vi "LabVIEW host computer v4.0.vi"() -> ()   [LabVIEW 2018]
uses:
  <vilib>/Instr/_visa.llb/VISA Configure Serial Port (Instr).vi
  <vilib>/regexp/Match Regular Expression.xnode
panel:
  out "HydrogenRemoteData":string="INSERT INTO MonitoringData(time, temperature, humidity)\nVALUES('2020/10/9 17:58:35', 24, 69)"
  in  "ConnectionString":string="DSN=myDB;"
  in  "选项卡控件":enum32{"双通道功率 ", "氢气浓度"}(tab)
  in  "选项卡控件 2":enum32{"通讯设置/数据显示"}(tab)
  in  "Reset":bool
  out "?":string
  in  "VISA resource name":refnum<visa-resource-name> caption="选择串口"
  in  "baud rate (9600)":u32=9600 caption="波特率"
  out "CH1 power":dbl
  out "?":string
  out "CH2 power":dbl
  out "CH1/CH2":dbl
  out "氢气浓度 4":dbl
  out "CH1 Power 2":dbl(graph)
  out "CH2 Power 2":dbl(graph)
  out "氢气浓度":dbl(graph)
  out "氢气浓度":dbl[](graph)
  in  "氢气输入":dbl[](array[numeric])
  out "氢气变化波长":dbl
  out "氢气浓度 3":dbl
  out "标定X":dbl[](array[numeric])
  out "氢气浓度 2":dbl
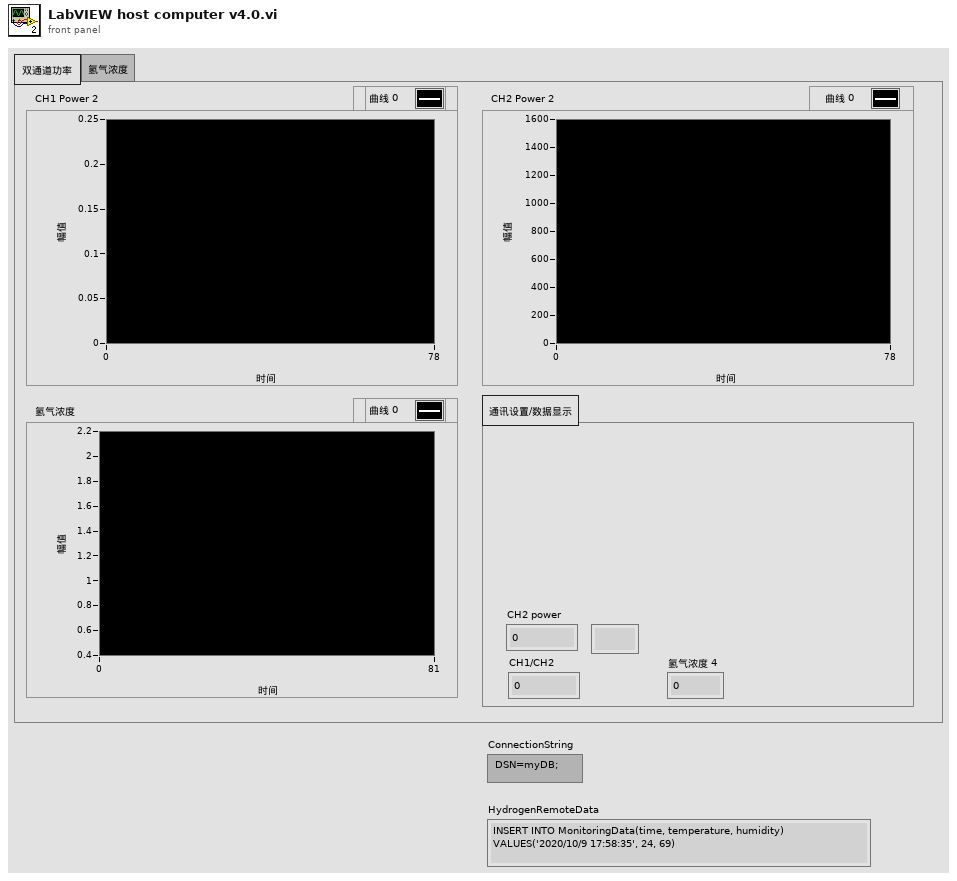
[diagram p1: front panel]
types:
  T1 = enum16{"open", "replace", "create", "open or create", "replace or create", "replace or create with confirmation"}
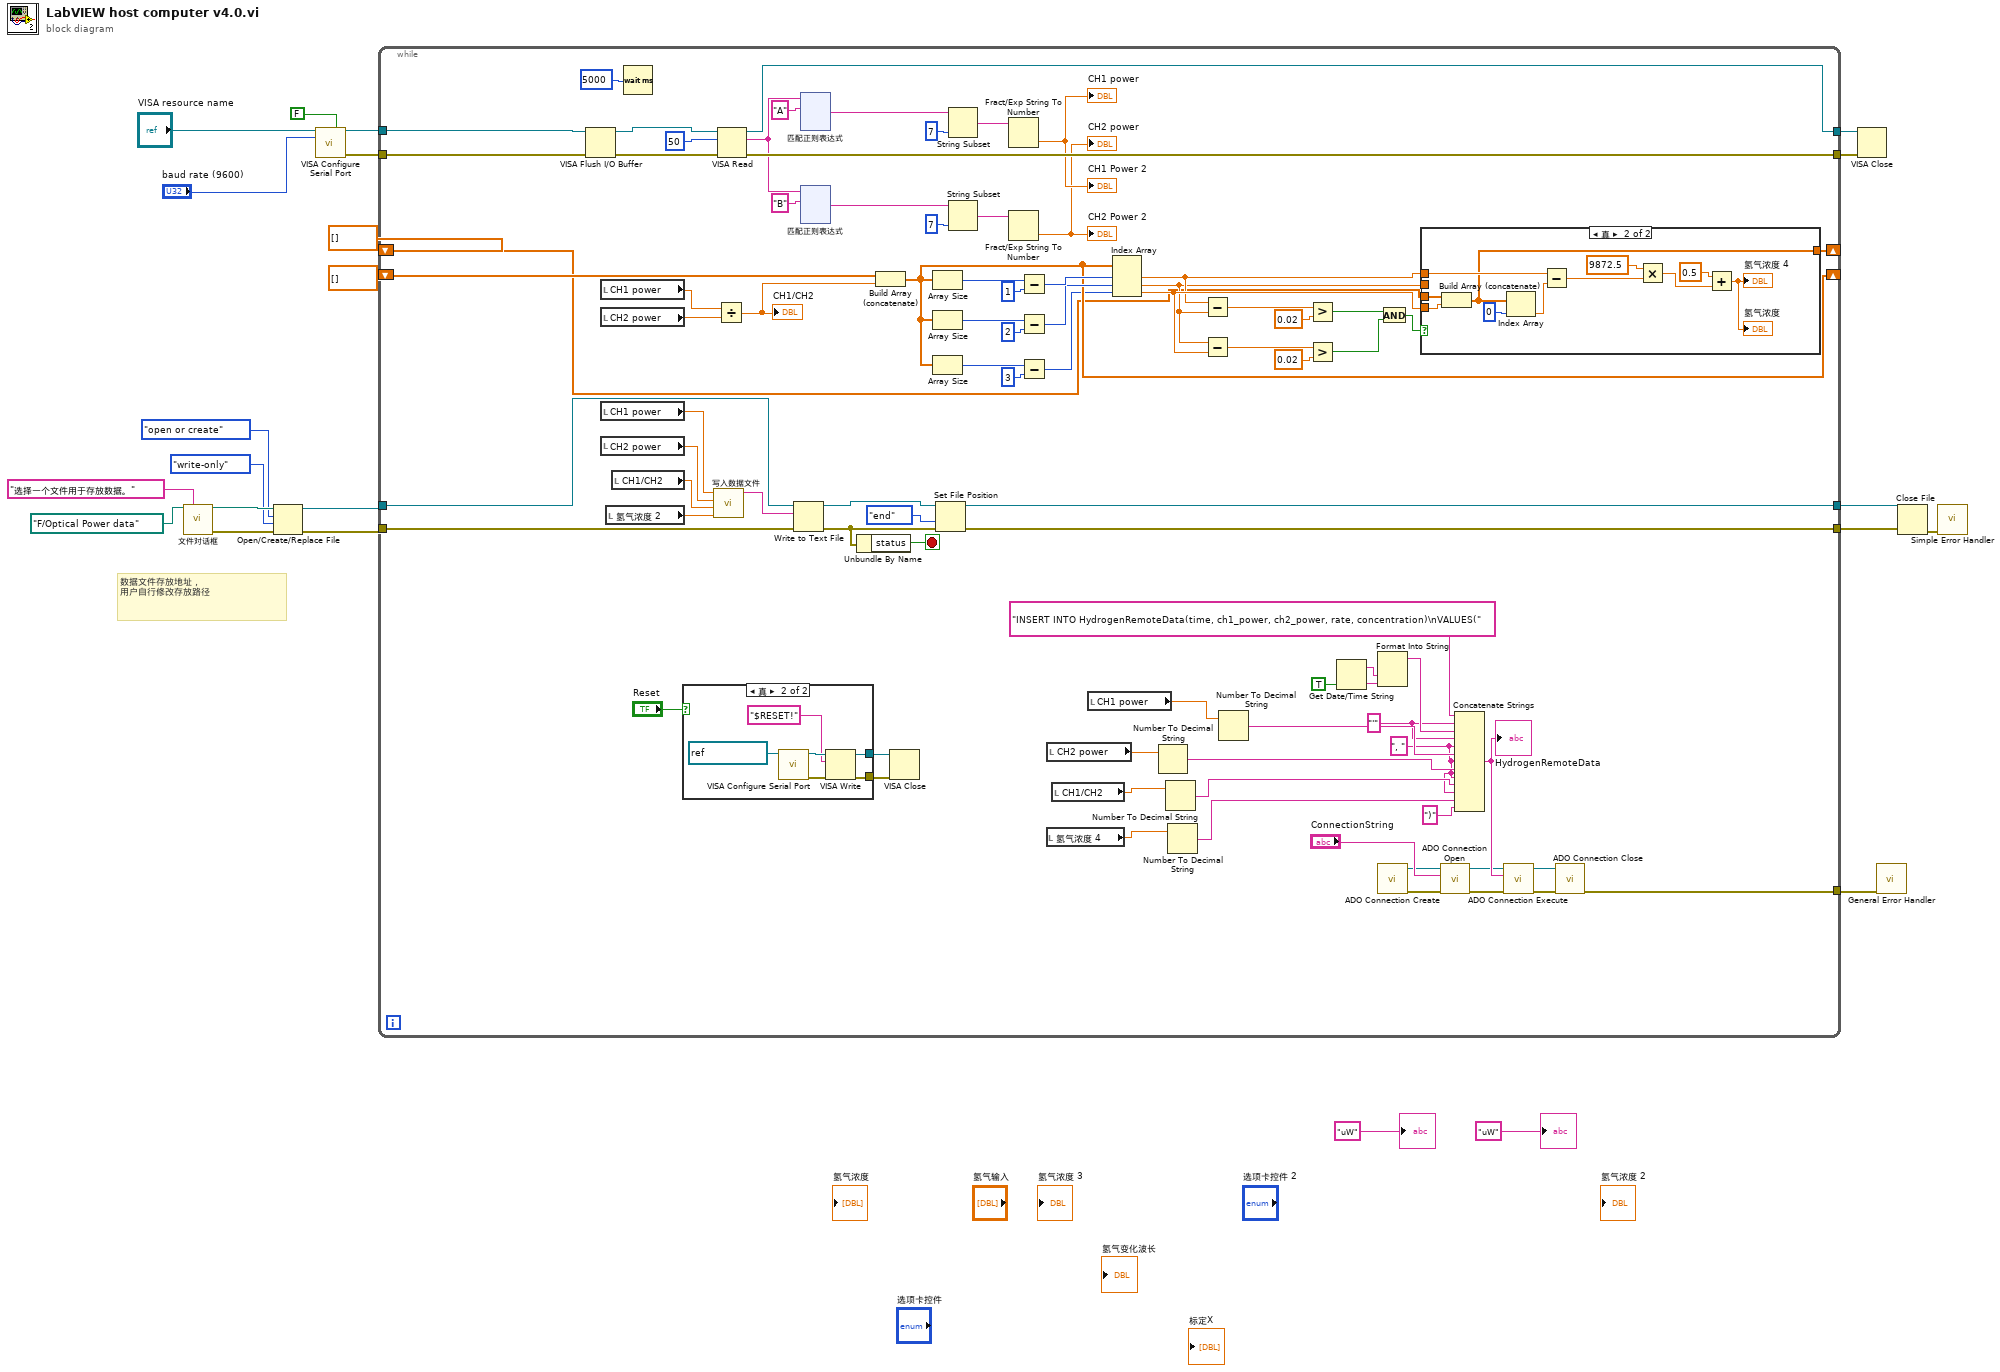
[diagram p0: block diagram]
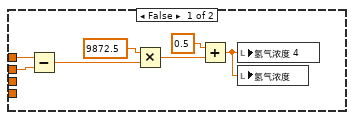
[diagram p3: hidden frame]
diagram:
  # "数据文件存放地址，\n用户自行修改存放路径"
  n1 = call "文件对话框"("start path"=path "F:/Optical Power data", "prompt"="选择一个文件用于存放数据。") -> ("selected path"=w15:path, "error out"=w14:errorcluster)  [unwired: 10 in, 2 out]
  n2 = Open/Create/Replace File(file path (use dialog)=w15, error in=w14, operation (0:open)=T1."open or create" ("操作(0:open)"), access (0:read/write)=enum16{"read/write", "read-only", "write-only"}."write-only" ("权限(0:read/write)")) -> (refnum out=w10:refnum<file>, error out=w9:errorcluster)  [unwired: 2 in, 1 out]
  n3 = call-poly "VISA Configure Serial Port"("VISA resource name"="VISA resource name", "Enable Termination\nChar (T)"=FALSE ("Enable Termination\nChar (T)"), "baud rate (9600)"="baud rate (9600)") -> ("VISA resource name out"=w20:refnum<visa-resource-name>, "error out"=w19:errorcluster)  [unwired: 11 in]
  n4 = while {
    tunnel: w20 -> [w108]
    tunnel: w19 -> [w107]
    tunnel: [w104] -> w18
    tunnel: w10 -> [w88]
    tunnel: w9 -> [w87]
    tunnel: [w86] -> w8
    tunnel: [w85] -> w7
    tunnel: [w84] -> w6
    shift-right: [w63] -> _
    shift-left: dbl[] [] -> [w68]
    shift-right: [w52] -> _
    shift-left: dbl[] [] -> [w53]
    tunnel: [w24] -> w1
    stop <- w89 stop-if-true
    w28 = ", " ("字符串")
    w34 = "'" ("字符串")
    n5 = VISA Flush I/O Buffer(VISA resource name=w108, error in (no error)=w107) -> (VISA resource name out=w106:refnum<visa-resource-name>, error out=w105:errorcluster)  [unwired: 1 in]
    n6 = local read "CH1 power"() -> (w78:dbl)
    n7 = local read "CH2 power"() -> (w77:dbl)
    n8 = local read "CH1 power"() -> (w93:dbl)
    n9 = local read "CH2 power"() -> (w94:dbl)
    n10 = local read "氢气浓度 2"() -> (w96:dbl)
    n11 = local read "CH1/CH2"() -> (w95:dbl)
    n12 = Wait (ms)(milliseconds to wait=u32 5000 ("毫秒计时值")) -> ()  [unwired: 1 out]
    n13 = case shown="真" "Reset" {
      tunnel: [_ w112] -> w50
      tunnel: [_ w111] -> w49
      frame False {
      }
      frame True {
        n14 = call-poly "VISA Configure Serial Port"("VISA resource name"=refnum<visa-resource-name> "COM3") -> ("VISA resource name out"=w114:refnum<visa-resource-name>, "error out"=w110:errorcluster)  [unwired: 13 in]
        n15 = VISA Write(VISA resource name=w114, write buffer="$RESET!" ("写入缓冲区"), error in (no error)=w110) -> (VISA resource name out=w112:refnum<visa-resource-name>, error out=w111:errorcluster)  [unwired: 1 out]
      }
    }
    n16 = call "写入数据文件.vi"("氢气浓度 2"=w96, "CH1/CH2"=w95, "CH2 Power"=w94, "CH1 Power"=w93) -> ("连接的字符串"=w97:string)  [unwired: 7 in]
    n17 = Divide(x=w78, y=w77) -> (x/y=w69:dbl)
    "CH1/CH2" <- w69
    n18 = VISA Read(VISA resource name=w106, byte count=u32 50 ("字节总数"), error in (no error)=w105) -> (VISA resource name out=w86:refnum<visa-resource-name>, read buffer=w83:string, error out=w104:errorcluster)  [unwired: 1 out]
    n19 = Write to Text File(file (use dialog)=w88, text=w97, error in=w87) -> (refnum out=w90:refnum<file>, error out=w91:errorcluster)  [unwired: 1 in, 1 out]
    n20 = xnode "匹配正则表达式"("输入字符串"=w83, "正则表达式"="A") -> ("匹配之后"=w102:string)  [unwired: 4 in, 4 out]
    n21 = xnode "匹配正则表达式"("输入字符串"=w83, "正则表达式"="B") -> ("匹配之后"=w98:string)  [unwired: 4 in, 4 out]
    n22 = Unbundle By Name(w91) -> ("status"=w89:bool)
    n23 = Build Array (concatenate)(w68, w69) -> (w63:dbl[])
    n24 = VISA Close(VISA resource name=w50, error in (no error)=w49) -> ()  [unwired: 1 out]
    n25 = Array Size(array=w63) -> (size(s)=w75:i32)
    n26 = Array Size(array=w63) -> (size(s)=w72:i32)
    n27 = Array Size(array=w63) -> (size(s)=w65:i32)
    n28 = Set File Position(refnum=w90, from (0:start)=enum16{"start", "end", "current"}."end" ("自（0:起始）"), error in=w91) -> (refnum out=w85:refnum<file>, error out=w84:errorcluster)  [unwired: 1 in]
    n29 = String Subset(string=w102, length (rest)=7 ("长度（剩余）")) -> (substring=w82:string)  [unwired: 1 in]
    n30 = String Subset(string=w98, length (rest)=7 ("长度（剩余）")) -> (substring=w80:string)  [unwired: 1 in]
    n31 = Fract/Exp String To Number(string=w82) -> (number=→"CH1 Power 2" →"CH1 power":dbl)  [unwired: 3 in, 1 out]
    n32 = Fract/Exp String To Number(string=w80) -> (number=→"CH2 Power 2" →"CH2 power":dbl)  [unwired: 3 in, 1 out]
    n33 = Subtract(x=w75, y=1) -> (x-y=w73:i32)
    n34 = Subtract(x=w72, y=2) -> (x-y=w70:i32)
    n35 = Subtract(x=w65, y=3) -> (x-y=w62:i32)
    n36 = local read "氢气浓度 4"() -> (w27:dbl)
    n37 = local read "CH2 power"() -> (w31:dbl)
    n38 = local read "CH1/CH2"() -> (w30:dbl)
    n39 = local read "CH1 power"() -> (w32:dbl)
    n40 = Index Array(array=w63, index #1=w73, index #2=w70, index #3=w62) -> (element #1=w55:dbl, element #2=w54:dbl, element #3=w56:dbl)
    n41 = Number To Decimal String(number=w31) -> (decimal integer string=w36:string)  [unwired: 1 in]
    n42 = Number To Decimal String(number=w30) -> (decimal integer string=w29:string)  [unwired: 1 in]
    n43 = Number To Decimal String(number=w27) -> (decimal integer string=w26:string)  [unwired: 1 in]
    n44 = Subtract(x=w55, y=w54) -> (x-y=w67:dbl)
    n45 = Subtract(x=w54, y=w56) -> (x-y=w60:dbl)
    n46 = Number To Decimal String(number=w32) -> (decimal integer string=w45:string)  [unwired: 1 in]
    n47 = Greater?(x=w67, y=0.02) -> (0:w59:bool)
    n48 = Greater?(x=w60, y=0.02) -> (0:w58:bool)
    n49 = Get Date/Time String(want seconds? (F)=TRUE ("需要秒？(F)")) -> (date string=w48:string, time string=w47:string)  [unwired: 2 in]
    n50 = Format Into String(w48, w47) -> (resulting string=w46:string)  [unwired: 3 in, 1 out]
    n51 = call <userlib>:"ADO Connection Create.vi"() -> ("error out"=w40:errorcluster, "ADODB._Connection Out"=w37:refnum<k7>)  [unwired: 10 in]
    n52 = And(x=w59, y=w58) -> (x .and. y?=w57:bool)
    n53 = case shown="真" w57 {
      tunnel: w56 -> [_ w127]
      tunnel: w55 -> [w122 w133]
      tunnel: w54 -> [w121 _]
      tunnel: w53 -> [_ w124]
      tunnel: [_ w123] -> w52
      frame False {
        n54 = Subtract(x=w122, y=w121) -> (x-y=w117:dbl)
        n55 = Multiply(x=9872.5, y=w117) -> (x*y=w119:dbl)
        n56 = Add(x=0.5, y=w119) -> (x+y=w116:dbl)
        n57 = local write "氢气浓度 4"(w116) -> ()
        n58 = local write "氢气浓度"(w116) -> ()
      }
      frame True {
        n59 = Build Array (concatenate)(w124, w127) -> (w123:dbl[])
        n60 = Index Array(array=w123, index=0 ("索引")) -> (element=w125:dbl)
        n61 = Subtract(x=w133, y=w125) -> (x-y=w132:dbl)
        n62 = Multiply(x=9872.5, y=w132) -> (x*y=w130:dbl)
        n63 = Add(x=0.5, y=w130) -> (x+y=→"氢气浓度 4" →"氢气浓度":dbl)
      }
    }
    n64 = call <userlib>:"ADO Connection Open.vi"("error in (no error)"=w40, "ConnectionString"="ConnectionString", "ADODB._Connection In"=w37) -> ("error out"=w41:errorcluster, "ADODB._Connection Out"=w38:refnum<k7>)  [unwired: 7 in]
    n65 = Concatenate Strings("INSERT INTO HydrogenRemoteData(time, ch1_power, ch2_power, rate, concentration)\nVALUES(", w34, w46, w34, w28, w45, w28, w36, w28, w29, w28, w26, ")" ("字符串")) -> (w44:string)
    "HydrogenRemoteData" <- w44
    n66 = call <userlib>:"ADO Connection Execute.vi"("error in (no error)"=w41, "CommandText"=w44, "ADODB._Connection In"=w38) -> ("error out"=w42:errorcluster, "ADODB._Connection Out"=w39:refnum<k7>)  [unwired: 6 in, 1 out]
    n67 = call <userlib>:"ADO Connection Close.vi"("error in (no error)"=w42, "ADODB._Connection In"=w39) -> ("error out"=w24:errorcluster)  [unwired: 8 in, 1 out]
  }
  n68 = VISA Close(VISA resource name=w8, error in (no error)=w18) -> ()  [unwired: 1 out]
  n69 = call <vilib>:"General Error Handler.vi"("error in (no error)"=w1) -> ()  [unwired: 10 in, 5 out]
  n70 = Close File(refnum=w7, error in=w6) -> (error out=w11:errorcluster)  [unwired: 1 out]
  n71 = call <vilib>:"Simple Error Handler.vi"("error in (no error)"=w11) -> ()  [unwired: 4 in, 5 out]
  "?" <- "uW"
  "?" <- "uW"
